vi "header data string.vi"(9 "Timing Control Parameters":T1 {"Measurment time interval" format="%.2e"}, 10 "N temps":i32, 11 "Temperature Control Parameters":T2 {"End Temp" format="%.2f"; "Temp Step" format="%.2f"; "Start Temp" format="%.2f"}) -> (3 "Concatenated String":string)   [LabVIEW 2014]
doc: "this vi creates a string for the data file header using the control parameters.\n\nPaul K Dixon\nPhysics 350\nCSUSB Physics"
panel:
  # "Header Data String Generator"
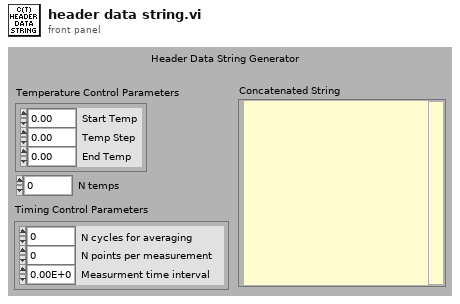
[diagram p1: front panel]
types:
  T1 = cluster{"N cycles for averaging":i32, "N points per measurement":i32, "Measurment time interval":dbl}
  T2 = cluster{"Start Temp":dbl, "Temp Step":dbl, "End Temp":dbl}
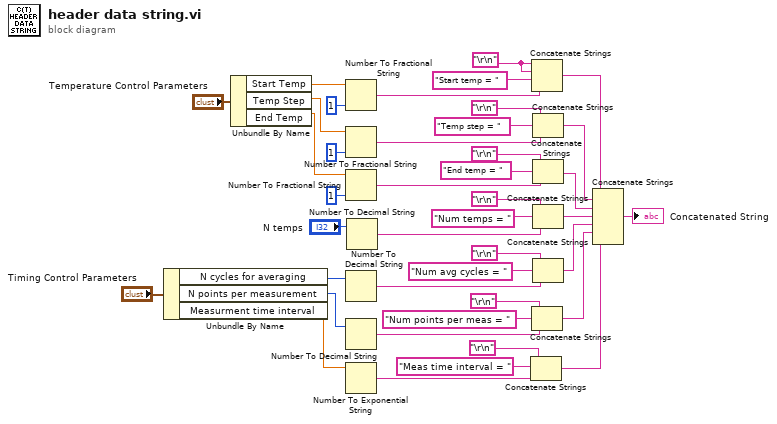
[diagram p0: block diagram]
diagram:
  w10 = "\r\n"
  n1 = Unbundle By Name("Timing Control Parameters") -> ("N cycles for averaging"=w5:i32, "N points per measurement"=w4:i32, "Measurment time interval"=w3:dbl)
  n2 = Unbundle By Name("Temperature Control Parameters") -> ("Start Temp"=w1:dbl, "Temp Step"=w2:dbl, "End Temp"=w7:dbl)
  n3 = Number To Fractional String(number=w1, precision (6)=i16 1) -> (F-format string=w40:string)  [unwired: 2 out]
  n4 = Number To Fractional String(number=w2, precision (6)=i16 1) -> (F-format string=w39:string)  [unwired: 2 out]
  n5 = Number To Fractional String(number=w7, precision (6)=i16 1) -> (F-format string=w38:string)  [unwired: 2 out]
  n6 = Number To Decimal String(number=w5) -> (decimal integer string=w36:string)  [unwired: 1 out]
  n7 = Number To Decimal String(number=w4) -> (decimal integer string=w35:string)  [unwired: 1 out]
  n8 = Number To Exponential String(number=w3) -> (E-format string=w34:string)  [unwired: 3 out]
  n9 = Number To Decimal String(number="N temps") -> (decimal integer string=w37:string)  [unwired: 1 out]
  n10 = Concatenate Strings("\r\n", "Meas time interval = ", w34) -> (w11:string)
  n11 = Concatenate Strings(w10, w10, "Start temp = ", w40) -> (w17:string)
  n12 = Concatenate Strings("\r\n", "Num points per meas = ", w35) -> (w12:string)
  n13 = Concatenate Strings("\r\n", "Temp step = ", w39) -> (w16:string)
  n14 = Concatenate Strings("\r\n", "End temp = ", w38) -> (w15:string)
  n15 = Concatenate Strings("\r\n", "Num temps = ", w37) -> (w14:string)
  n16 = Concatenate Strings("\r\n", "Num avg cycles = ", w36) -> (w13:string)
  n17 = Concatenate Strings(w17, w16, w15, w14, w13, w12, w11) -> (→"Concatenated String":string)
